vi "FixPixmapColourArraySize.vi"(8 "error in (no error)":errorcluster, 11 "image data in":T1) -> (0 "error out":errorcluster, 3 "image data out":T1)   [LabVIEW 2020, in "g_ar_toolkit.image.lvlib"]
uses:
  g_ar_toolkit.image.lvlib
  <vilib>/picture/picture.llb/imagedata.ctl
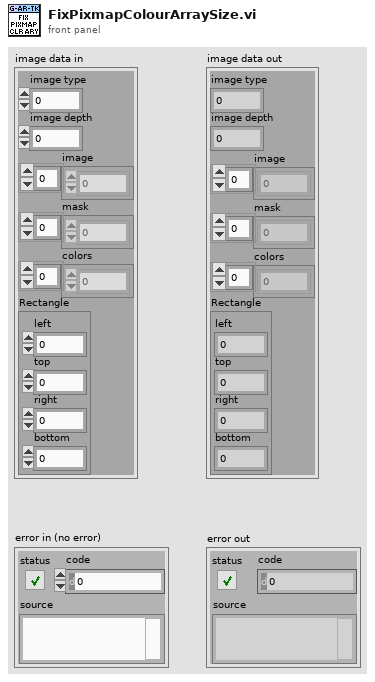
[diagram p1: front panel]
types:
  T1 = typedef "imagedata.ctl" = cluster{"image type":i32, "image depth":i32, "image":u8[], "mask":u8[], "colors":u32[], "Rectangle":cluster{"left":i16, "top":i16, "right":i16, "bottom":i16}}
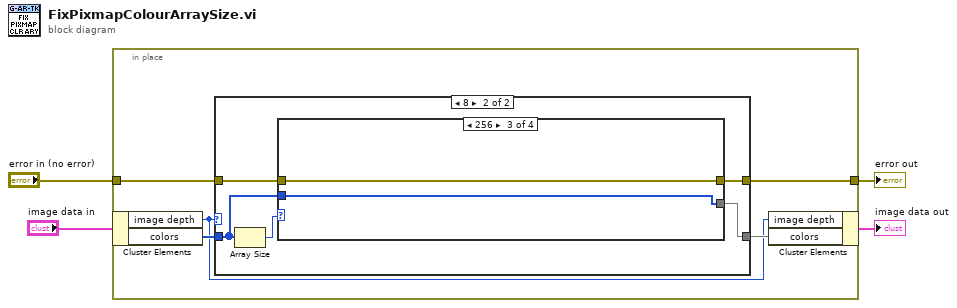
[diagram p0: block diagram]
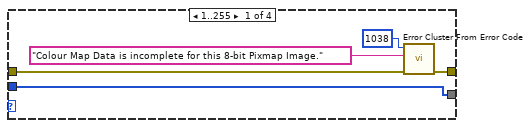
[diagram p3: hidden frame]
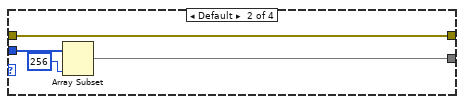
[diagram p4: hidden frame]
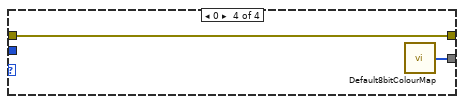
[diagram p5: hidden frame]
diagram:
  n1 = in-place {
    in-place-border: "error in (no error)" -> [w6]
    in-place-border: [w5] -> w1
    n2 = in-place-cluster #1("image data in") -> ("image depth"=w7:i32, "colors"=w9:u32[])
    n3 = case shown="8" w7 {
      tunnel: w9 -> [w11 w14]
      tunnel: [w11 w15] -> w8
      tunnel: w6 -> [w10 w13]
      tunnel: [w10 w12] -> w5
      frame Default {
      }
      frame 8 {
        n4 = Array Size(array=w14) -> (size(s)=w16:i32)
        n5 = case shown="256" w16 {
          tunnel: [w21 w24 w27 w29] -> w15
          tunnel: w14 -> [w21 w25 w27 _]
          tunnel: w13 -> [w20 w22 w26 w28]
          tunnel: [w17 w22 w26 w28] -> w12
          frame 1..255 {
            n6 = call <vilib>:"Error Cluster From Error Code.vi"("error in (no error)"=w20, "error message (\"\")"="Colour Map Data is incomplete for this 8-bit Pixmap Image." ("error message (\"\")"), "error code (0)"=1038) -> ("error out"=w17:errorcluster)  [unwired: 6 in]
          }
          frame Default {
            n7 = Array Subset(array=w25, length=256 ("x")) -> (w24:u32[])  [unwired: 1 in]
          }
          frame 256 {
          }
          frame 0 {
            n8 = call "Default8bitColourMap.vi"() -> ("Default 8-bit Colour Map"=w29:u32[])
          }
        }
      }
    }
    n9 = in-place-cluster #1("image depth"=w7, "colors"=w8) -> (→"image data out":T1)
  }
  "error out" <- w1
